vi "GetTerminals from node.vi"(8 "error in (no error)":errorcluster, 11 "Node":refnum<vi>) -> (0 "error out":errorcluster, 2 "Not Source Terminals[]":refnum<vi>[](array[refnum]), 3 "Source Terminals":refnum<vi>[](array[refnum]))   [LabVIEW 2014]
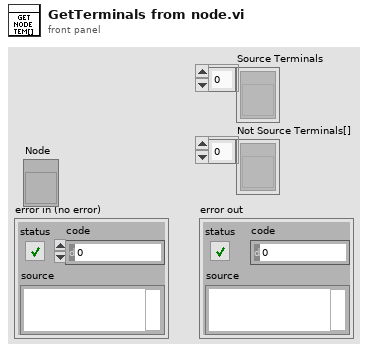
[diagram p1: front panel]
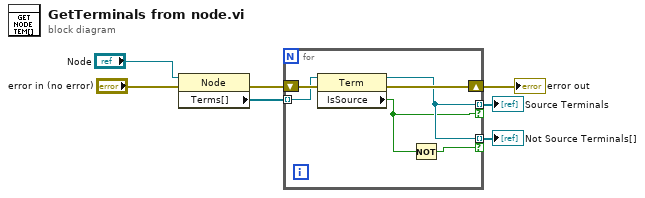
[diagram p0: block diagram]
diagram:
  n1 = property class="Node"(reference="Node", error in="error in (no error)") -> (error out=w5:errorcluster, "Terms[]"=w3:refnum<vi>[])  [unwired: 1 out]
  n2 = for {
    tunnel: w3 -> [w11] mode=indexing
    shift-right: [w12] -> w4
    shift-left: w5 -> [w13]
    tunnel: [w10] -> w2 mode=indexing if=w8
    tunnel: [w10] -> w1 mode=indexing if=w9
    n3 = property class="Term"(reference=w11, error in=w13) -> (reference out=w10:refnum<vi>, error out=w12:errorcluster, "IsSource"=w8:bool)
    n4 = Not(x=w8) -> (.not. x?=w9:bool)
  }
  "error out" <- w4
  "Source Terminals" <- w2
  "Not Source Terminals[]" <- w1
